vi "ILABR_ViStatus.vi"(2 "port":i32, 3 "machineName":string, 4 "name":string) -> (0 "errorOut":string, 1 "status":i32)   [LabVIEW 2009]
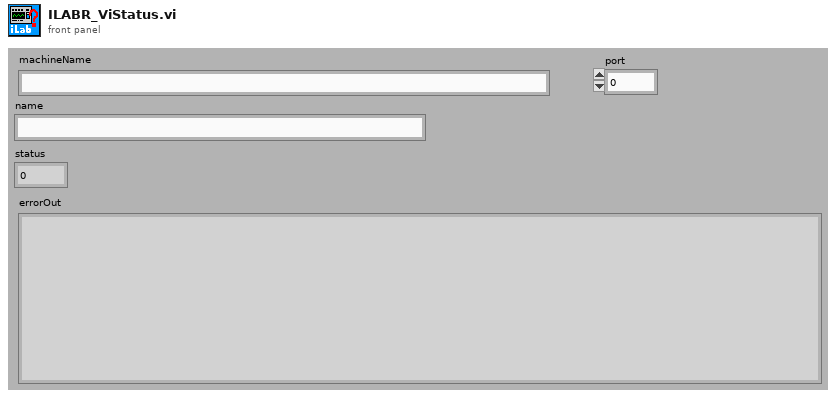
[diagram p1: front panel]
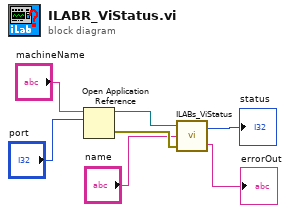
[diagram p0: block diagram]
diagram:
  n1 = Open Application Reference(10:"port", 11:"machineName") -> (0:w5:errorcluster, 3:w6:refnum<vi>)  [unwired: 1 in, 1 out]
  n2 = call "ILABs_ViStatus.vi"("errorIn"=w5, "name"="name", "appReference"=w6) -> ("errorOut"=→"errorOut":string, "status"=→"status":i32)
